vi "MainGUI.vi"(0 "reference in":refnum<class "TraceWindow.lvclass">, 5 "Error In":errorcluster) -> (14 "reference out":refnum<class "TraceWindow.lvclass">, 19 "Error Out":errorcluster)   [LabVIEW 2021, in "TraceWindow.lvlib" / "TraceWindow.lvclass"]
doc: "This template is based off of the Queued Message Handler design pattern and the Queued Message Handler project template that ships with LabVIEW.\n\nThe main difference is that the queue is private to this module and communication between modules is performed via Broadcast and Request events.\n\nRequest events are wrapped in public API methods and are handled in the Event Handling Loop (EHL) of this VI. Any module can register for Broadcast events sent by this module. The EHL generates messages based on user interface actions.\n\nThe Message Handling Loop (MHL) processes messages generated by the EHL, or by other messages. The messages are string values, so new messages can be added easily to the Message Cases case structure in the MHL. Each message cluster can also provide an optional value for Message Data, which is a variant that can be converted to whatever message-specific data is required.\n_____\nBased on Delacor QMH Project Template 4.2.0.63.\n\n<b>Note:</b> This VI was modified by the <b>Validate DQMH Module</b> tool to have the module name be passed as the Additional Information parameter with an Error Reported broadcast.\n\n<b>Note:</b> This VI was modified by the <b>Validate DQMH Module</b> tool to call the Release Message Queue VI in the top-level Error case."
uses:
  TraceWindow.lvclass
  TraceWindow_MessageData.ctl
  <vilib>/Utility/miscctls.llb/LVRowAndColumnUnsignedTypeDef.ctl
panel:
  out "Trace":string[][](table)
  out "Last Command":string
  in  "Size":i32=1000 format="%d lines"
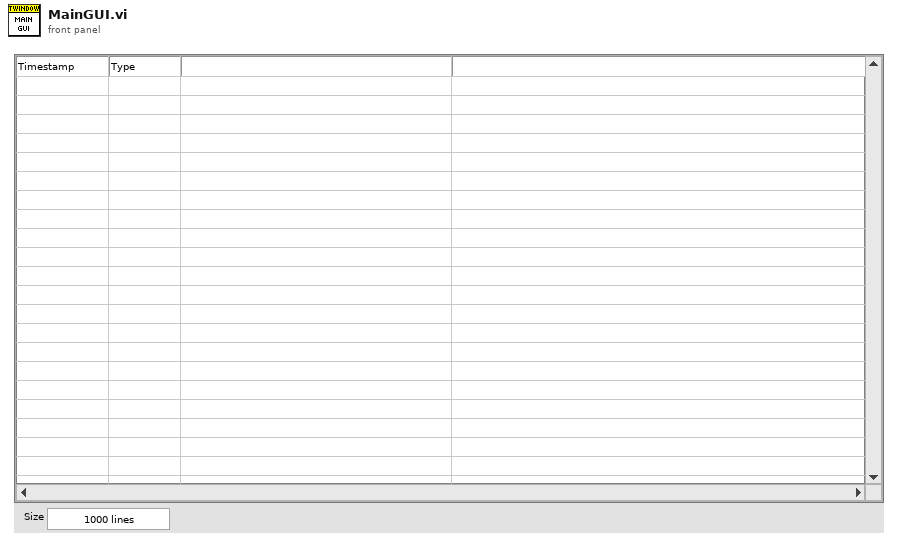
[diagram p1: front panel]
types:
  T1 = typedef "TraceWindow.lvlib/TraceWindow.lvclass/TraceWindow_MessageData.ctl" = cluster{"Show":cluster{"Send":cluster{"State":bool}, "Receive":cluster{"Dummy":bool}}, "WriteTraceQueue":cluster{"Send":cluster{"TraceQueue":refnum<queue>}, "Receive":cluster{"Dummy":bool}}}
  T2 = cluster{"Event":refnum<event-registration>, "Command":string, "MessageData":T1, "ReplyQueue":refnum<queue>, "TraceQueue":refnum<queue>}
  T3 = cluster{"ReplyQueue":refnum<queue>, "Data":variant}
  T4 = enum32{"Invalid", "Standard", "Closed", "Hidden", "Minimized", "Maximized"}
  T5 = typedef "LVRowAndColumnUnsignedTypeDef.ctl" = cluster{"Row":u32, "Column":u32}
  T6 = typedef "TraceWindow.lvlib/TraceWindow.lvclass/ObjectAttributes.ctl" = cluster{"Interfaces":cluster{"Dummys":refnum<class>}, "Locals":cluster{"MainGUIActive":refnum<queue>, "TraceQueue":refnum<queue>}, "Persistent":cluster{"OpenAtClosure":bool, "BufferSize":i32, "Startup":cluster{"OpenAtStartUp":bool, "OpenMinimized":bool}}}
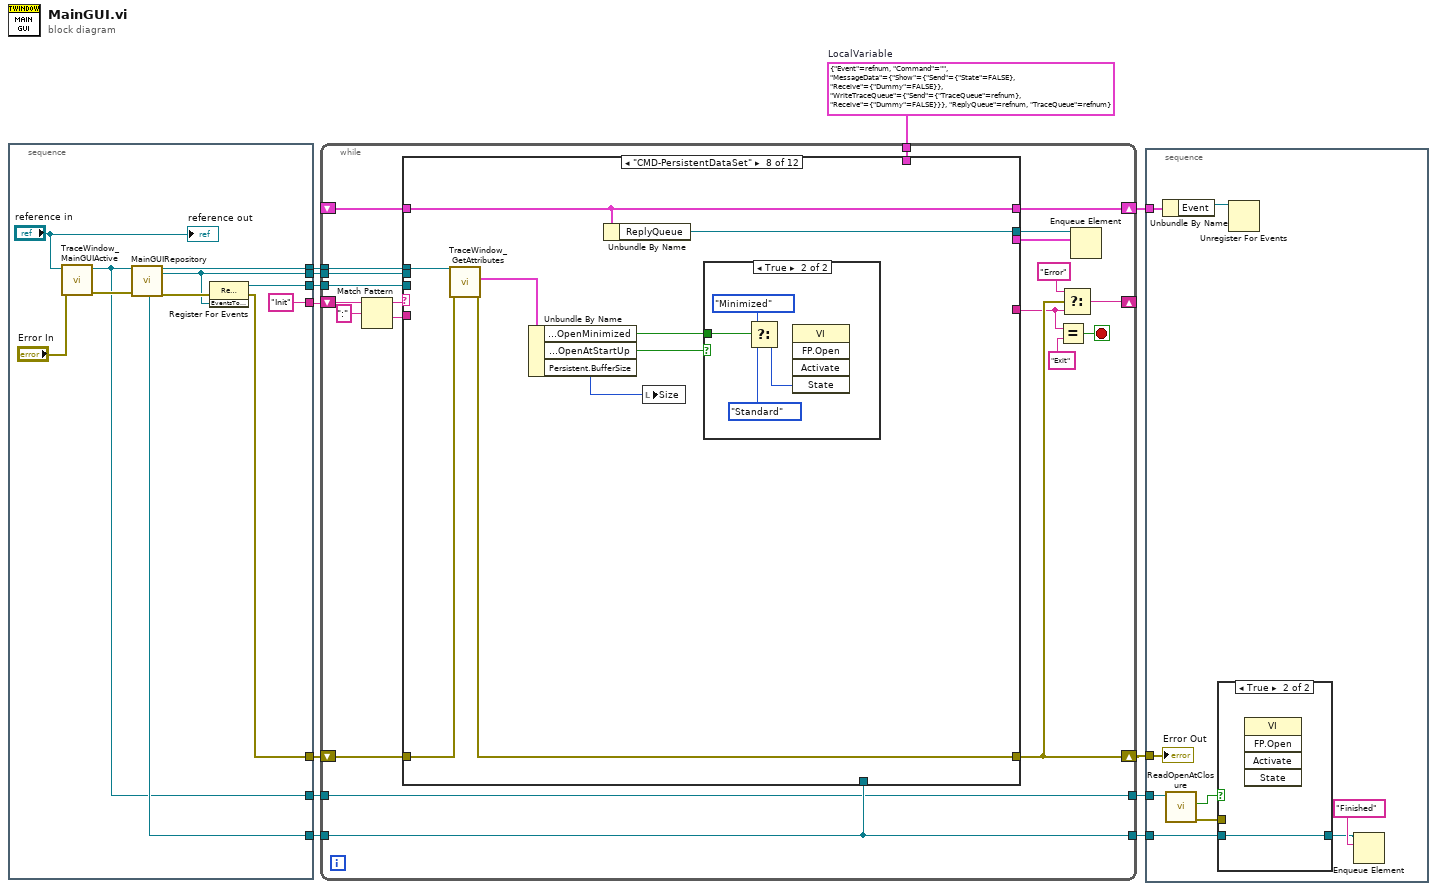
[diagram p0: block diagram]
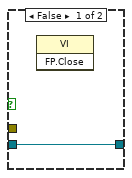
[diagram p2: hidden frame]
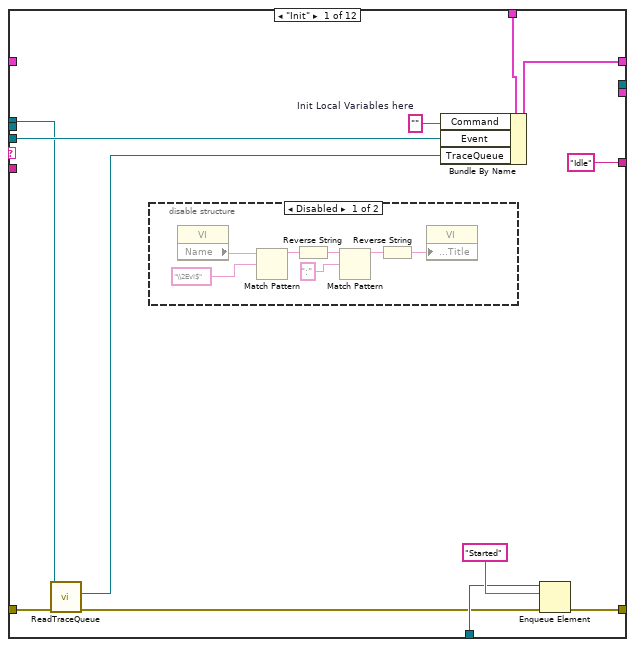
[diagram p3: hidden frame]
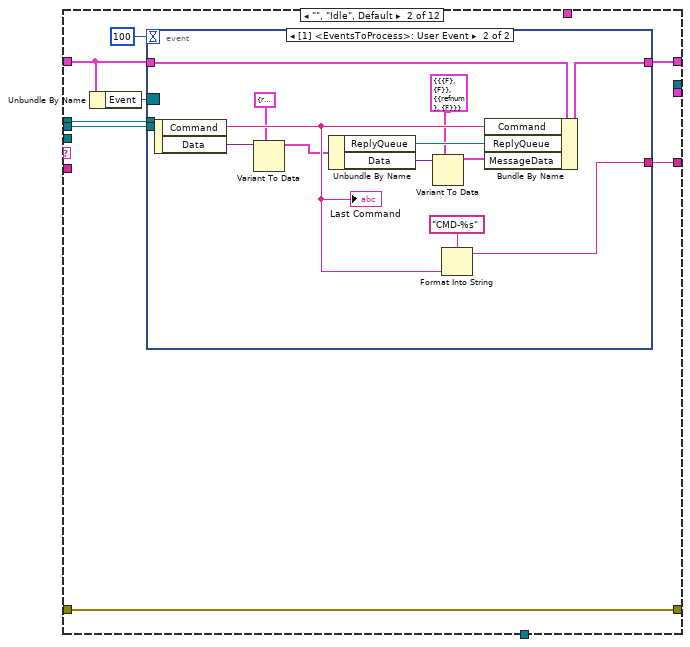
[diagram p5: hidden frame]
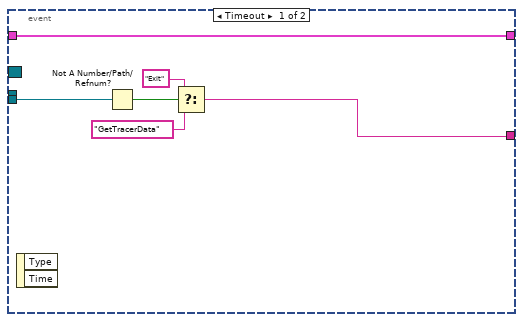
[diagram p6: hidden frame]
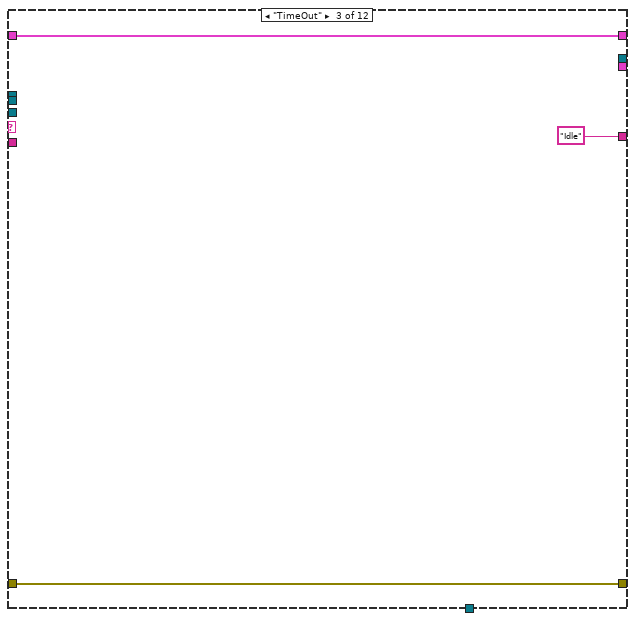
[diagram p7: hidden frame]
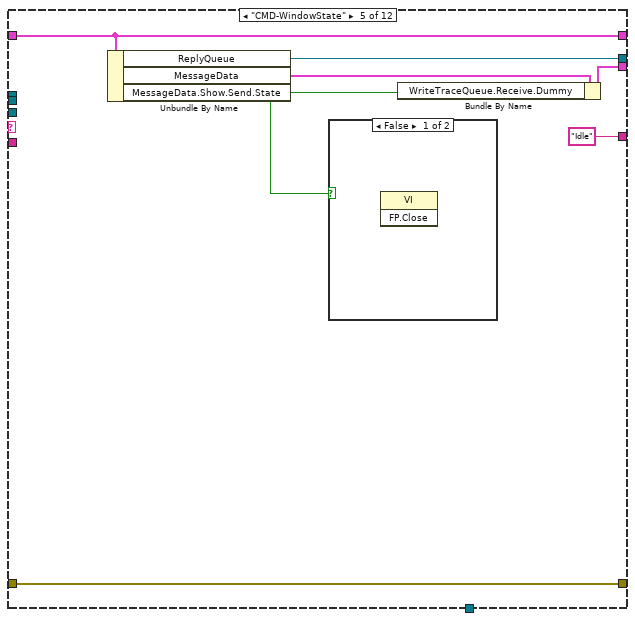
[diagram p9: hidden frame]
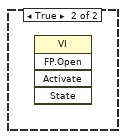
[diagram p10: hidden frame]
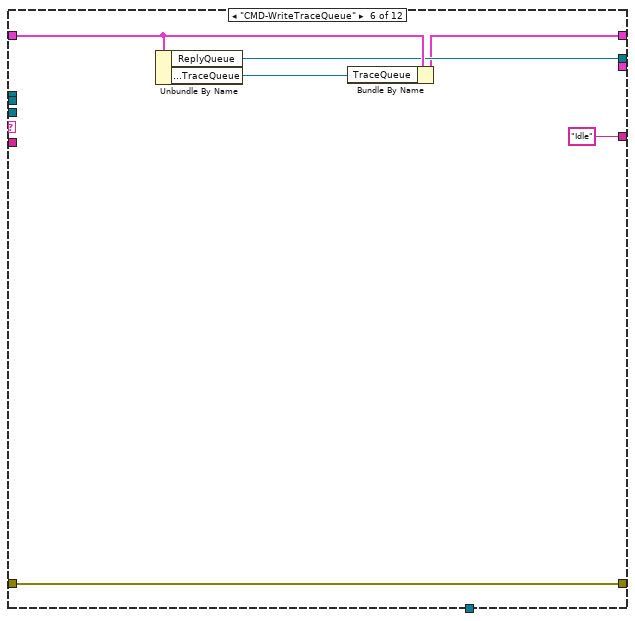
[diagram p11: hidden frame]
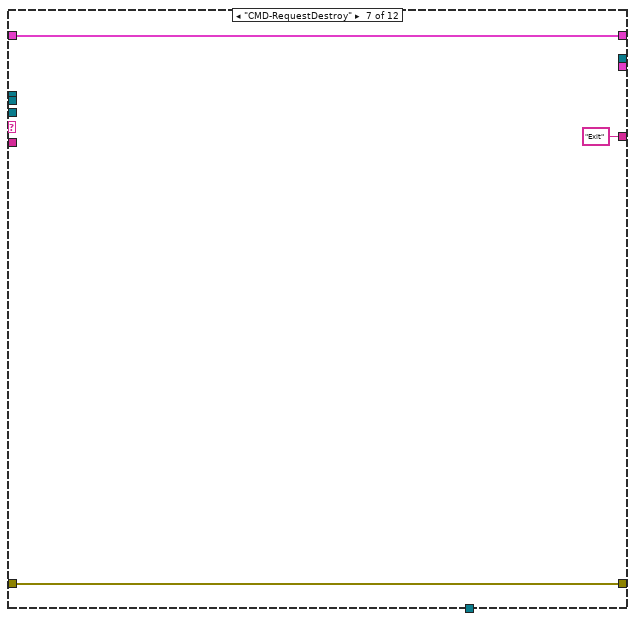
[diagram p12: hidden frame]
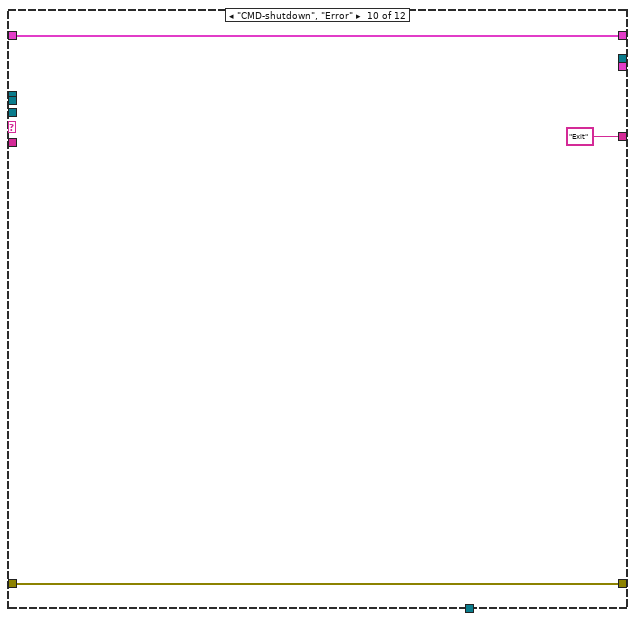
[diagram p15: hidden frame]
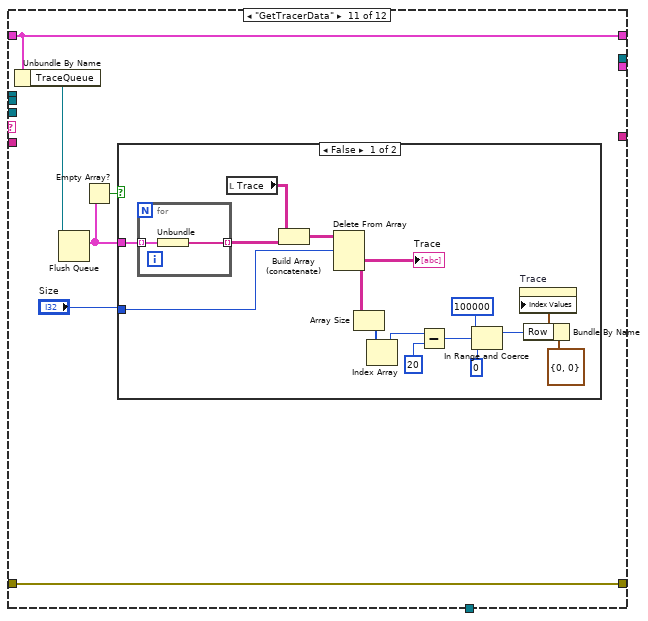
[diagram p16: hidden frame]
diagram:
  w7 = T2 {"Event"=refnum, "Command"="", "MessageData"={"Show"={"Send"={"State"=FALSE}, "Receive"={"Dummy"=FALSE}}, "WriteTraceQueue"={"Send"={"TraceQueue"=refnum}, "Receive"={"Dummy"=FALSE}}}, "ReplyQueue"=refnum, "TraceQueue"=refnum}  # LocalVariable
  n1 = stacked-sequence {
    tunnel: [w17] -> w12
    tunnel: [w23] -> w10
    tunnel: [w20] -> w9
    tunnel: ["Init"] -> w8
    tunnel: [w18] -> w5
    tunnel: [w15] -> w3
    tunnel: [w13] -> w2
    frame #0 {
      n2 = call "TraceWindow_MainGUIActive.vi"("Error In"="Error In", "reference in"="reference in") -> ("Error Out"=w14:errorcluster, "reference out"=w13:refnum<class "TraceWindow.lvclass">)  [unwired: 8 in]
      n3 = call "MainGUIRepository.vi"("reference in"=w13, "Error In"=w14) -> ("ProcessSyncQueue"=w18:refnum<queue>, "reference out"=w23:refnum<class "TraceWindow.lvclass">, "EventsToProcess"=w15:refnum<user-event>, "Error Out"=w19:errorcluster)  [unwired: 10 in, 4 out]
      n4 = register-events(error in=w19, w15) -> (reference out=w20:refnum<event-registration>, error out=w17:errorcluster)  [unwired: 1 in]
      "reference out" <- "reference in"
    }
  }
  n5 = while {
    shift-right: [w37] -> w11
    shift-left: w12 -> [w42]
    tunnel: w10 -> [w43]
    tunnel: w9 -> [w44]
    shift-right: [w35] -> _
    shift-left: w8 -> [w40]
    shift-right: [w31] -> w6
    shift-left: _ -> [w30]
    tunnel: w7 -> [w29]
    tunnel: [w26] -> w4
    tunnel: w5 -> [w26]
    tunnel: w3 -> [w25]
    tunnel: [w24] -> w1
    tunnel: w2 -> [w24]
    stop <- w32 stop-if-true
    n6 = Match Pattern(string=w40, regular expression=":") -> (before substring=w39:string, after substring=w38:string)  [unwired: 1 in, 2 out]
    n7 = case shown="\"CMD-PersistentDataSet\"" w39 {
      tunnel: w42 -> [w47 w66 w92 w94 w101 w107 w110 w116 w125 w128 w134 w153]
      tunnel: [w50 w66 w92 w94 w101 w107 w110 w117 w125 w128 w134 w153] -> w37
      tunnel: w44 -> [w52 _ _ _ _ _ _ _ _ _ _ _]
      tunnel: w43 -> [w46 w65 _ _ _ _ _ w119 _ _ _ _]
      tunnel: w38 -> [_ _ _ _ _ _ _ _ _ _ _ _]
      tunnel: ["Idle" ("t") w71 "Idle" ("t") _ "Idle" ("t") "Idle" ("t") "Exit" ("y") _ _ "Exit" ("y") _ _] -> w34
      tunnel: [w56 w70 w90 w93 w99 w103 w109 w113 w124 w126 w131 w152] -> w31
      tunnel: w30 -> [_ w69 w90 w93 w99 w105 w109 w113 w124 w126 w131 w152]
      tunnel: w29 -> [w53 _ _ _ _ _ _ _ _ _ _ _]
      tunnel: [_ _ _ _ w98 w104 _ w112 _ _ _ _] -> w28
      tunnel: [_ _ _ _ w96 _ _ _ _ _ _ _] -> w27
      tunnel: w26 -> [w49 _ _ _ _ _ _ _ _ _ _ _]
      tunnel: w25 -> [_ w64 _ _ _ _ _ _ _ _ _ _]
      frame "Init" {
        w55 = ""  # Init Local Variables here
        n8 = call-dynamic "ReadTraceQueue.vi"("Error In"=w47, "reference in"=w46) -> ("Error Out"=w48:errorcluster, "TraceQueue"=w45:refnum<queue>)  [unwired: 7 in, 1 out]
        n9 = disable-structure shown="Disabled" {
          frame Disabled {
            n10 = property class="VI"() -> ("Name"=w63:string)  [unwired: 2 in, 2 out]
            n11 = Match Pattern(string=w63, regular expression="\\2Evi$") -> (before substring=w61:string)  [unwired: 1 in, 3 out]
            n12 = Reverse String(1:w61) -> (0:w60:string)
            n13 = Match Pattern(string=w60, regular expression=":") -> (before substring=w58:string)  [unwired: 1 in, 3 out]
            n14 = Reverse String(1:w58) -> (0:w57:string)
            n15 = property class="VI"("Front Panel.Title"=w57) -> ()  [unwired: 2 in, 2 out]
          }
          frame Enabled {
          }
        }
        n16 = Bundle By Name(cluster=w53, "Command"=w55, "Event"=w52, "TraceQueue"=w45) -> (w56:T2)
        n17 = Enqueue Element(queue=w49, element="Started", error in (no error)=w48) -> (error out=w50:errorcluster)  [unwired: 1 in, 2 out]
      }
      frame "", "Idle", Default {
        n18 = Unbundle By Name(w69) -> ("Event"=w68:refnum<event-registration>)
        n19 = event shown="[1] <EventsToProcess>: User Event" {
          selector: w68 -> [_ _]
          dyn-events: _ -> [_ _]
          timeout: 100 -> [_ _]
          tunnel: [w73 w86] -> w71
          tunnel: w69 -> [w72 w89]
          tunnel: [w72 w88] -> w70
          tunnel: w65 -> [_ _]
          tunnel: w64 -> [w74 _]
          event Timeout {
            n20 = event-data() -> ()  [unwired: 1 in, 2 out]
            n21 = Not A Number/Path/Refnum?(number/path/refnum=w74) -> (NaN/Path/Refnum?=w75:bool)
            n22 = Select(t="Exit", s=w75, f="GetTracerData" ("t")) -> (s? t:f=w73:string)
          }
          event User Event {
            n23 = event-data() -> ("Command"=w85:string, "Data"=w84:variant)  [unwired: 1 in]
            "Last Command" <- w85
            n24 = Variant To Data(type=T3 {"ReplyQueue"=refnum, "Data"=variant} ("output cluster"), Variant=w84) -> (data=w82:T3)  [unwired: 1 in, 1 out]
            n25 = Unbundle By Name(w82) -> ("ReplyQueue"=w81:refnum<queue>, "Data"=w80:variant)
            n26 = Variant To Data(type=T1 {"Show"={"Send"={"State"=FALSE}, "Receive"={"Dummy"=FALSE}}, "WriteTraceQueue"={"Send"={"TraceQueue"=refnum}, "Receive"={"Dummy"=FALSE}}} ("MessageData"), Variant=w80) -> (data=w79:T1)  [unwired: 1 in, 1 out]
            n27 = Format Into String(format string="CMD-%s", w85) -> (resulting string=w86:string)  [unwired: 2 in, 1 out]
            n28 = Bundle By Name(cluster=w89, "Command"=w85, "ReplyQueue"=w81, "MessageData"=w79) -> (w88:T2)
          }
        }
      }
      frame "TimeOut" {
      }
      frame "---- COMMANDS START----" {
      }
      frame "CMD-WindowState" {
        n29 = Unbundle By Name(w99) -> ("ReplyQueue"=w98:refnum<queue>, "MessageData"=w97:T1, "MessageData.Show.Send.State"=w95:bool)
        n30 = case shown="False" w95 {
          frame False {
            n31 = invoke class="VI" method="FP.Close"() -> ()  [unwired: 3 in, 3 out]
          }
          frame True {
            n32 = invoke class="VI" method="FP.Open"() -> ()  [unwired: 5 in, 5 out]
          }
        }
        n33 = Bundle By Name(cluster=w97, "WriteTraceQueue.Receive.Dummy"=w95) -> (w96:T1)
      }
      frame "CMD-WriteTraceQueue" {
        n34 = Unbundle By Name(w105) -> ("ReplyQueue"=w104:refnum<queue>, "MessageData.WriteTraceQueue.Send.TraceQueue"=w102:refnum<queue>)
        n35 = Bundle By Name(cluster=w105, "TraceQueue"=w102) -> (w103:T2)
      }
      frame "CMD-RequestDestroy" {
      }
      frame "CMD-PersistentDataSet" {
        n36 = call "TraceWindow_GetAttributes.vi"("error in (no error)"=w116, "reference in"=w119) -> ("error out"=w117:errorcluster, "Data"=w118:T6)  [unwired: 6 in, 2 out]
        n37 = Unbundle By Name(w118) -> ("Persistent.Startup.OpenMinimized"=w111:bool, "Persistent.Startup.OpenAtStartUp"=w115:bool, "Persistent.BufferSize"=w114:i32)
        n38 = Unbundle By Name(w113) -> ("ReplyQueue"=w112:refnum<queue>)
        n39 = local write "Size"(w114) -> ()
        n40 = case shown="True" w115 {
          tunnel: w111 -> [_ w123]
          frame False {
          }
          frame True {
            n41 = Select(t=T4."Minimized" ("State"), s=w123, f=T4."Standard" ("State")) -> (s? t:f=w120:T4)
            n42 = invoke class="VI" method="FP.Open"("State"=w120) -> ()  [unwired: 4 in, 5 out]
          }
        }
      }
      frame "----- COMMANDS END ----" {
      }
      frame "CMD-shutdown", "Error" {
      }
      frame "GetTracerData" {
        n43 = Unbundle By Name(w131) -> ("TraceQueue"=w130:refnum<queue>)
        n44 = Flush Queue(queue=w130) -> (remaining elements=w132:cluster{string[]}[])  [unwired: 1 in, 2 out]
        n45 = Empty Array?(array=w132) -> (empty?=w133:bool)
        n46 = case shown="False" w133 {
          tunnel: "Size" -> [w146 _]
          tunnel: w132 -> [w145 _]
          frame False {
            n47 = for {
              tunnel: w145 -> [w151] mode=indexing
              tunnel: [w150] -> w148 mode=indexing
              n48 = Unbundle(w151) -> (w150:string[])
            }
            n49 = local read "Trace"() -> (w149:string[][])
            n50 = Build Array (concatenate)(w149, w148) -> (w147:string[][])
            n51 = Delete From Array(array=w147, length=w146) -> (deleted portion=w135:string[][])  [unwired: 2 in, 1 out]
            "Trace" <- w135
            n52 = Array Size(array=w135) -> (size(s)=w142:i32[])
            n53 = Index Array(array=w142) -> (element=w141:i32)  [unwired: 1 in]
            n54 = Subtract(x=w141, y=20) -> (x-y=w137:i32)
            n55 = In Range and Coerce(upper limit=100000, x=w137, lower limit=0) -> (coerced(x)=w140:i32)  [unwired: 1 out]
            n56 = Bundle By Name(cluster=T5 {"Row"=0, "Column"=0} ("Index Values"), "Row"=w140) -> (w143:T5)
            n57 = property on="Trace" class="Tbl (strict)"("Index Values"=w143) -> ()  [unwired: 2 in, 2 out]
          }
          frame True {
          }
        }
      }
      frame "----- UI ACTIONS -----" {
      }
    }
    n58 = Equal?(x=w34, y="Exit") -> (x = y?=w32:bool)
    n59 = Select(t="Error", s=w37, f=w34) -> (s? t:f=w35:string)
    n60 = Enqueue Element(queue=w28, element=w27) -> ()  [unwired: 2 in, 3 out]
  }
  n61 = stacked-sequence {
    tunnel: w11 -> [w162]
    tunnel: w4 -> [w158]
    tunnel: w6 -> [w161]
    tunnel: w1 -> [w156]
    frame #0 {
      n62 = Unbundle By Name(w161) -> ("Event"=w160:refnum<event-registration>)
      n63 = call-dynamic "ReadOpenAtClosure.vi"("reference in"=w156) -> ("Error Out"=w154:errorcluster, "AutoClose"=w155:bool)  [unwired: 8 in, 1 out]
      n64 = case shown="True" w155 {
        tunnel: [w163 w164] -> w157
        tunnel: w158 -> [w163 w164]
        tunnel: w154 -> [_ _]
        frame False {
          n65 = invoke class="VI" method="FP.Close"() -> ()  [unwired: 3 in, 3 out]
        }
        frame True {
          n66 = invoke class="VI" method="FP.Open"() -> ()  [unwired: 5 in, 5 out]
        }
      }
      n67 = Unregister For Events(event registration refnum=w160) -> ()  [unwired: 1 in, 1 out]
      n68 = Enqueue Element(queue=w157, element="Finished") -> ()  [unwired: 2 in, 3 out]
      "Error Out" <- w162
    }
  }
